vi "Test DI and DO.vi"() -> ()   [LabVIEW 2013]
uses:
  SLL DAQ Engine/Software/Source Code/Sub VIs/DAQ Engine/Controls/SLL DE List of Digital Inputs.ctl
  SLL DAQ Engine/Software/Source Code/Sub VIs/DAQ Engine/Controls/SLL DE List of Digital Outputs.ctl
  SLL DAQ Engine/Software/Source Code/Sub VIs/DAQ Engine/Controls/SLL DE DI Global Options.ctl
  SLL DAQ Engine/Software/Source Code/Sub VIs/DAQ Engine/Controls/SLL DE DO Global Options.ctl
panel:
  out "DO Channel Name":T1
  out "String":string
  in  "PC_ACK_Read_Tags":dbl
  in  "Invalid_SNo":dbl
  in  "Station_No_Start_Stop_Test":dbl
  in  "Start_Test":dbl
  in  "Rerun":dbl
  in  "Station_Number":dbl
  in  "Test_Result":dbl
  in  "Serial_Flange_Size":string
  in  "Serial_Displacement_Size":dbl
  in  "Serial_Adapter_Size":dbl
  in  "New_Serial":dbl
  in  "Scan_Trigger":dbl
  in  "Stop_Test":dbl
  in  "Task_Available_for_Robot":dbl
  in  "Robot_Available":dbl
  in  "DI Array":bool[](array[boolean])=[FALSE, FALSE, FALSE, FALSE, FALSE, FALSE, FALSE, FALSE, FALSE, FALSE, FALSE, FALSE, FALSE, FALSE, FALSE, FALSE, FALSE, FALSE, FALSE, FALSE, FALSE, FALSE, FALSE, FALSE, FALSE, FALSE, FALSE, FALSE]
  in  "DI Channel Name Array":T2[](array[typedef])=[enum."STATION1_START", enum."STATION1_STOP", enum."STATION1_CLAMPED", enum."STATION1_TC_PASS", enum."STATION1_TC_FAIL", enum."STATION1_TTA", enum."STATION1_TTB", enum."STATION2_START", enum."STATION2_STOP", enum."STATION2_CLAMPED", enum."STATION2_TC_PASS", enum."STATION2_TC_FAIL", enum."STATION2_TTA", enum."STATION2_TTB", enum."STATION3_START", enum."STATION3_STOP", enum."STATION3_CLAMPED", enum."STATION3_TC_PASS", enum."STATION3_TC_FAIL", enum."STATION3_TTA", enum."STATION3_TTB", enum."STATION4_START", enum."STATION4_STOP", enum."STATION4_CLAMPED", enum."STATION4_TC_PASS", enum."STATION4_TC_FAIL", enum."STATION4_TTA", enum."STATION4_TTB"]
  out "DO Channel Name Array":T1[](array[typedef])=[enum."STATION1_START TEST", enum."STATION1_STOP TEST", enum."STATION1_LIGHT1", enum."STATION1_LIGHT2", enum."STATION1_LIGHT3", enum."STATION1_SELECT_TEST", enum."STATION2_START TEST", enum."STATION2_STOP TEST", enum."STATION2_LIGHT1", enum."STATION2_LIGHT2", enum."STATION2_LIGHT3", enum."STATION2_SELECT_TEST", enum."STATION3_START TEST", enum."STATION3_STOP TEST", enum."STATION3_LIGHT1", enum."STATION3_LIGHT2", enum."STATION3_LIGHT3", enum."STATION3_SELECT_TEST", enum."STATION4_START TEST", enum."STATION4_STOP TEST", enum."STATION4_LIGHT1", enum."STATION4_LIGHT2", enum."STATION4_LIGHT3", enum."STATION4_SELECT_TEST"]
  out "DO Status":bool[](array[boolean])
  out "error out":errorcluster
  in  "error in":errorcluster
  in  "DI Channel Name":T2
  in  "stop":bool
  # "Simulation VI to send DI Status and reads the DO output"
  # "Write Tags\nPC Writes to PLC\nPLC can only read these tags"
  # "Read Tags\nPC Reads from PLC"
  # "Test Type1: TTA:1, TTB: 0;\nTest Type2: TTA:0, TTB: 1;\nTest Type3: TTA:1, TTB: 1;\nTest Type4: TTA:0, TTB: 0;"
  # "IDLE : \t\t100\nTest Running:\t 010\nPass\t\t110\nFail\t\t101"
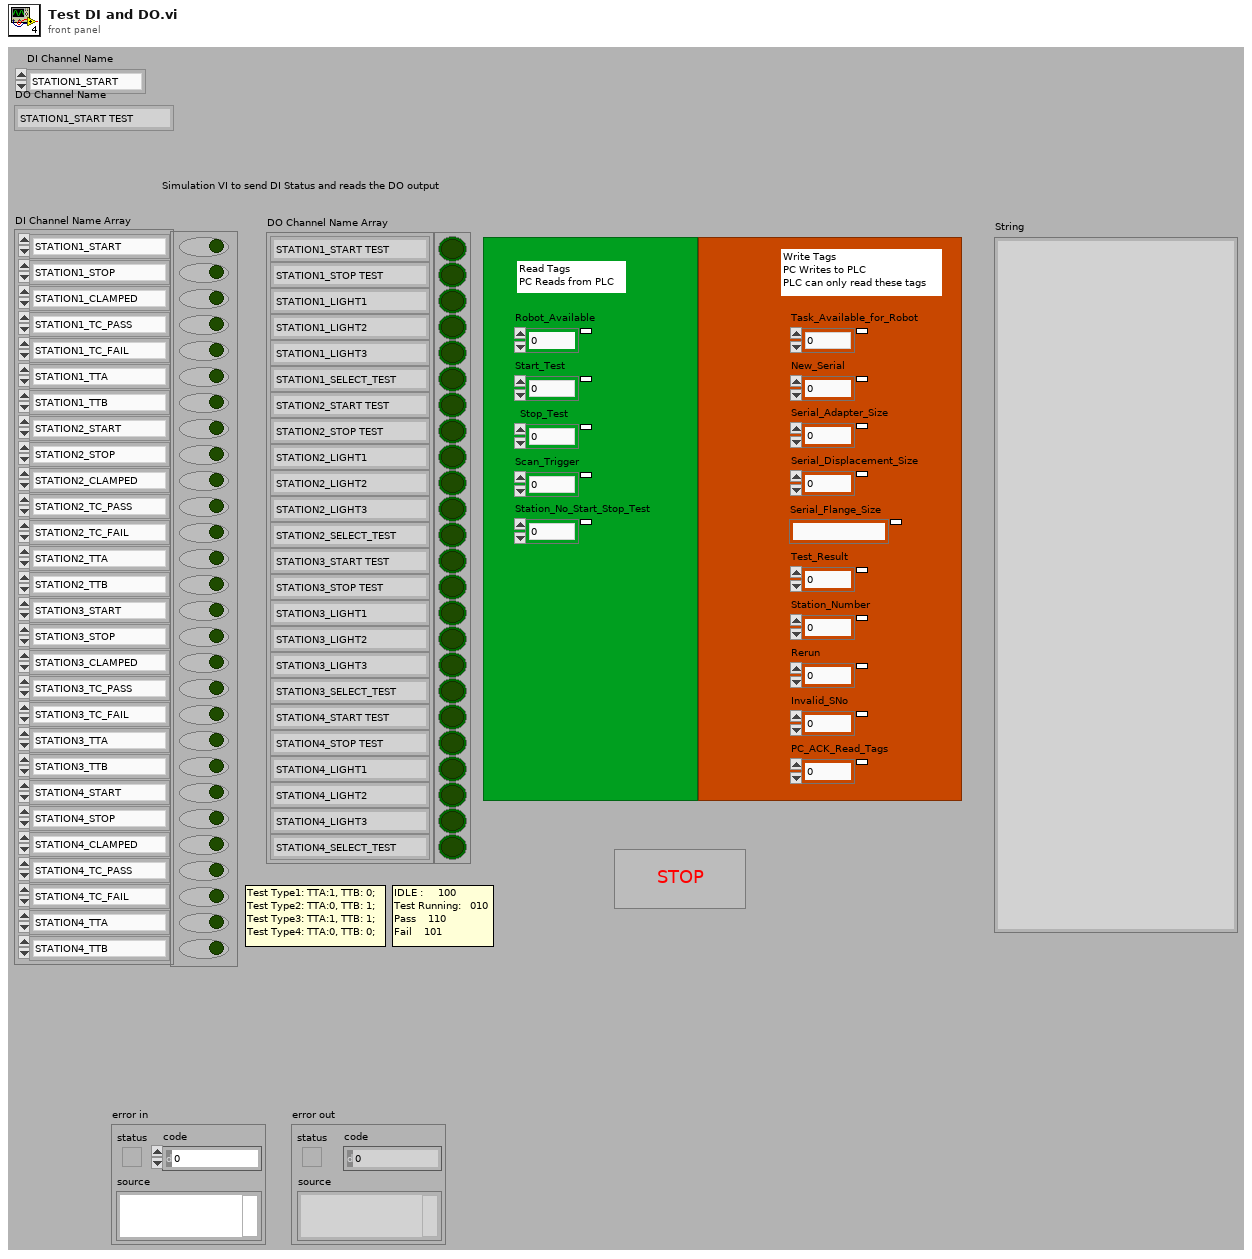
[diagram p1: front panel]
types:
  T1 = typedef "SLL DE List of Digital Outputs.ctl" = enum16{"STATION1_START TEST", "STATION1_STOP TEST", "STATION1_LIGHT1", "STATION1_LIGHT2", "STATION1_LIGHT3", "STATION1_SELECT_TEST", "STATION2_START TEST", "STATION2_STOP TEST", "STATION2_LIGHT1", "STATION2_LIGHT2", "STATION2_LIGHT3", "STATION2_SELECT_TEST", "STATION3_START TEST", "STATION3_STOP TEST", "STATION3_LIGHT1", "STATION3_LIGHT2", "STATION3_LIGHT3", "STATION3_SELECT_TEST", "STATION4_START TEST", "STATION4_STOP TEST", "STATION4_LIGHT1", "STATION4_LIGHT2", "STATION4_LIGHT3", "STATION4_SELECT_TEST"}
  T2 = typedef "SLL DE List of Digital Inputs.ctl" = enum16{"STATION1_START", "STATION1_STOP", "STATION1_CLAMPED", "STATION1_TC_PASS", "STATION1_TC_FAIL", "STATION1_TTA", "STATION1_TTB", "STATION2_START", "STATION2_STOP", "STATION2_CLAMPED", "STATION2_TC_PASS", "STATION2_TC_FAIL", "STATION2_TTA", "STATION2_TTB", "STATION3_START", "STATION3_STOP", "STATION3_CLAMPED", "STATION3_TC_PASS", "STATION3_TC_FAIL", "STATION3_TTA", "STATION3_TTB", "STATION4_START", "STATION4_STOP", "STATION4_CLAMPED", "STATION4_TC_PASS", "STATION4_TC_FAIL", "STATION4_TTA", "STATION4_TTB"}
  T3 = enum32{"No PSP", "Read", "Write", "Write & Read"}
  T4 = typedef "SLL DE DO Global Options.ctl" = enum16{"Init", "Write Line", "Write Array", "Write Full Status", "Read Line", "Read Array", "Read Full Status", "Restart DO", "Send to Safe Mode", "Stop DO"}
  T5 = typedef "SLL DE DI Global Options.ctl" = enum16{"Init", "Write Line", "Write Array", "Read Line", "Read Array", "Read Full Status", "Write Full Status"}
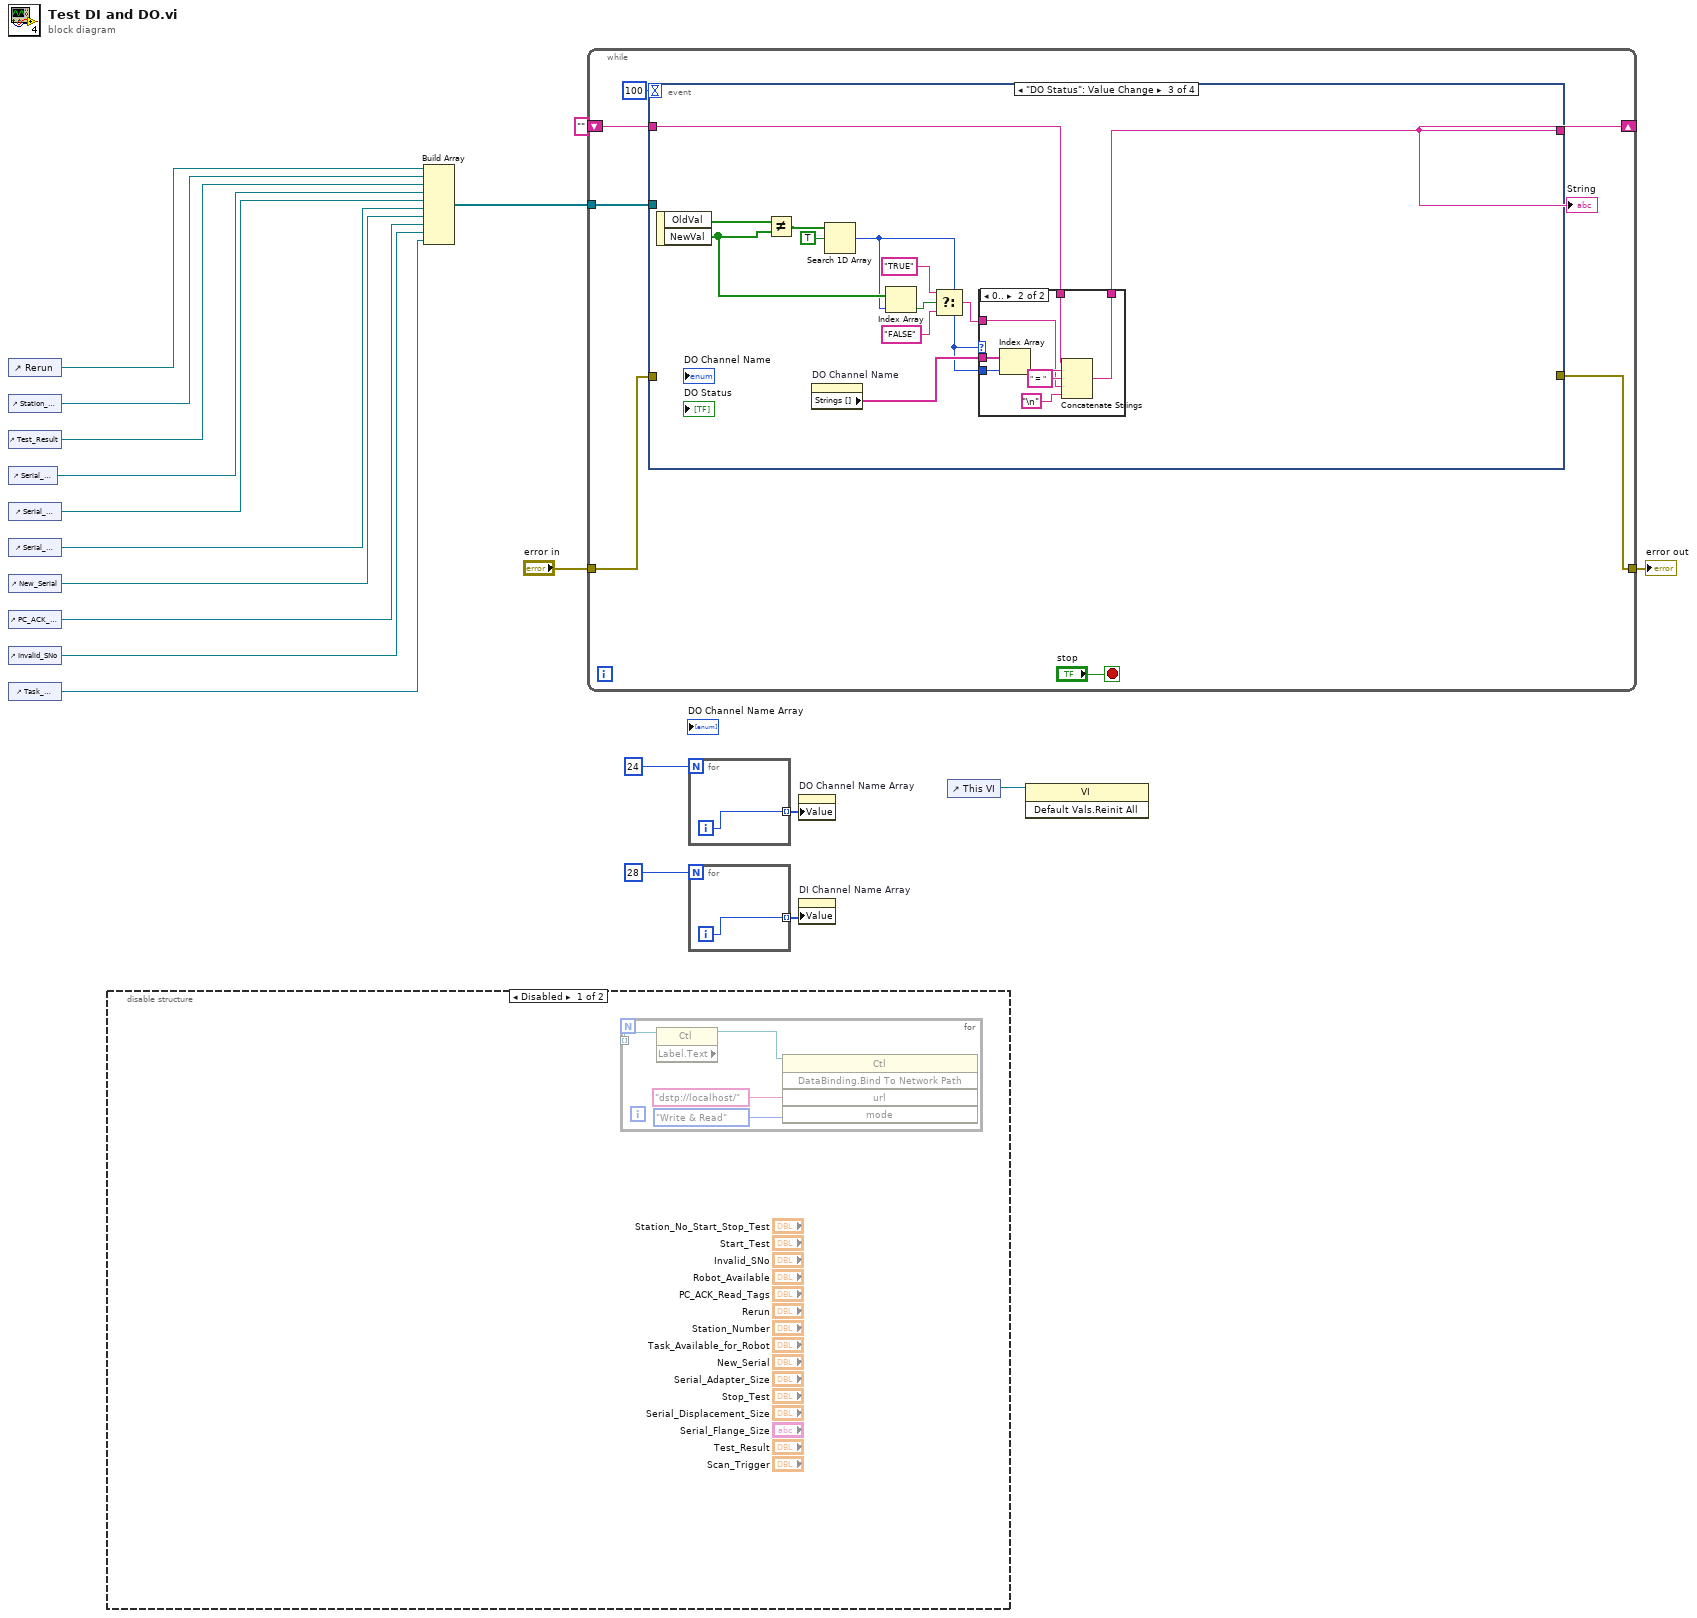
[diagram p0: block diagram]
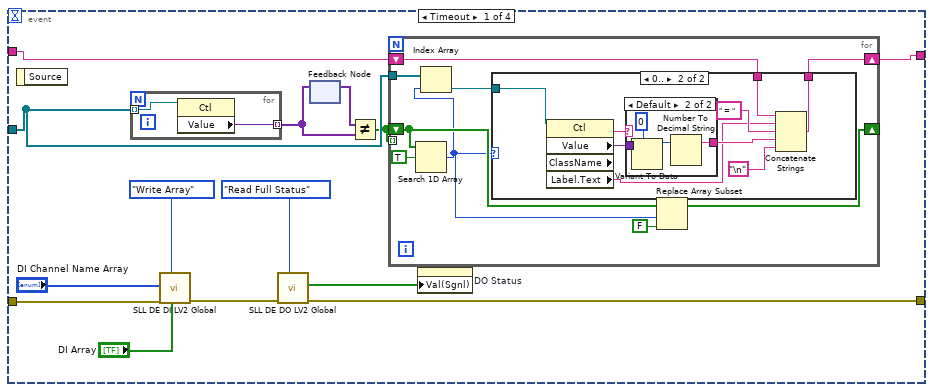
[diagram p3: hidden frame]
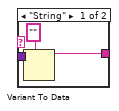
[diagram p5: hidden frame]
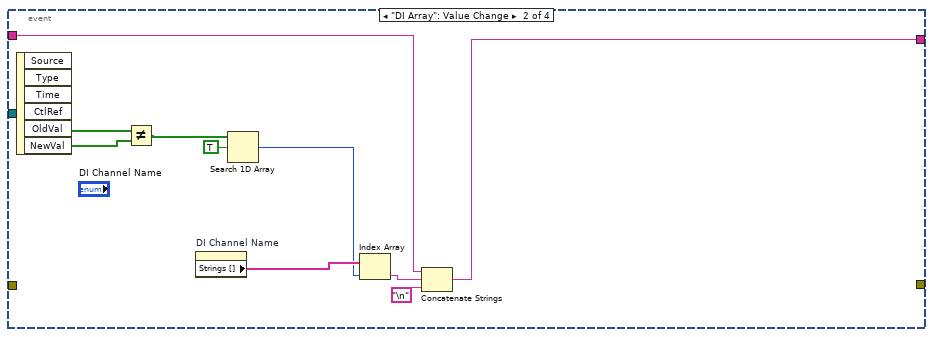
[diagram p6: hidden frame]
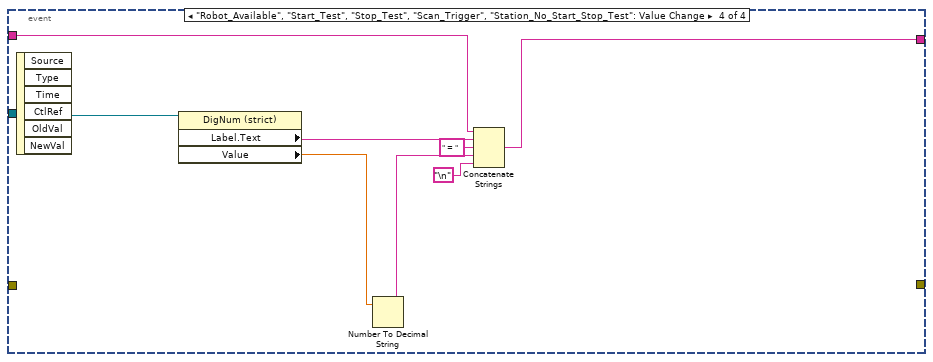
[diagram p8: hidden frame]
diagram:
  n1 = control-ref of="Rerun"() -> (w2:refnum<vi>)
  n2 = control-ref of="Station_Number"() -> (w3:refnum<vi>)
  n3 = control-ref of="Test_Result"() -> (w4:refnum<vi>)
  n4 = control-ref of="Serial_Flange_Size"() -> (w5:refnum<vi>)
  n5 = control-ref of="Serial_Displacement_Size"() -> (w6:refnum<vi>)
  n6 = control-ref of="Serial_Adapter_Size"() -> (w7:refnum<vi>)
  n7 = control-ref of="New_Serial"() -> (w8:refnum<vi>)
  n8 = control-ref of="PC_ACK_Read_Tags"() -> (w9:refnum<vi>)
  n9 = control-ref of="Invalid_SNo"() -> (w10:refnum<vi>)
  n10 = control-ref of="Task_Available_for_Robot"() -> (w11:refnum<vi>)
  n11 = disable-structure shown="Disabled" {
    frame Disabled {
      n12 = for {
        tunnel: [w24] -> w20 mode=indexing
        n13 = property class="Ctl" props=["Label", "Text"](reference=w24) -> (reference out=w21:refnum<vi>)  [unwired: 1 in, 2 out]
        n14 = invoke on="Invoke Node" class="Ctl" method="DataBinding.Bind To Network Path"(reference=w21, "url"="dstp://localhost/" ("URL"), "mode"=T3."Write & Read" ("Mode")) -> ()  [unwired: 2 in, 5 out]
      }
    }
    frame Enabled {
    }
  }
  n15 = Build Array(w2, w3, w4, w5, w6, w7, w8, w9, w10, w11) -> (w1:refnum<vi>[])
  n16 = while {
    tunnel: "error in" -> [w27]
    tunnel: [w26] -> w19
    shift-right: [w30] -> _
    shift-left: "" -> [w28]
    tunnel: w1 -> [w25]
    stop <- "stop" stop-if-true
    n17 = event shown="[2] \"DO Status\": Value Change" {
      selector: _ -> [_ _ _ _]
      dyn-events: _ -> [_ _ _ _]
      timeout: 100 -> [_ _ _ _]
      tunnel: [w33 w75 w92 w110] -> w30
      tunnel: w28 -> [w34 w74 w91 w111]
      tunnel: w27 -> [w39 _ _ _]
      tunnel: [w38 _ _ _] -> w26
      tunnel: w25 -> [w35 _ _ _]
      event Timeout {
        n18 = event-data() -> ()  [unwired: 1 in, 1 out]
        n19 = for {
          tunnel: w35 -> [w73] mode=indexing
          tunnel: [w72] -> w36 mode=indexing
          n20 = property class="Ctl"(reference=w73) -> ("Value"=w72:variant)  [unwired: 1 in, 2 out]
        }
        n21 = call "SLL DE DI LV2 Global.vi"("DI State Array"="DI Array", "Option"=SLL_DE_DI_Global_Options."Write Array", "error in (no error)"=w39, "DI Channel Name Array"="DI Channel Name Array") -> ("error out"=w44:errorcluster)  [unwired: 4 in, 3 out]
        n22 = call "SLL DE DO LV2 Global.vi"("DO Option"=SLL_DE_DO_Global_Options."Read Full Status", "Error In"=w44) -> ("error out"=w38:errorcluster, "Digital Array Status"=w45:bool[])  [unwired: 6 in, 2 out]
        n23 = feedback-in #1(w36) -> ()
        n24 = feedback #1() -> (w37:variant[])  [unwired: 1 in]
        n25 = Not Equal?(x=w37, y=w36) -> (x != y?=w32:bool[])
        n26 = for {
          tunnel: w35 -> [w53]
          shift-right: [w48] -> _
          shift-left: w32 -> [w49]
          tunnel: w32 -> [_] mode=indexing
          shift-right: [w51] -> w33
          shift-left: w34 -> [w52]
          n27 = Search 1D Array(1D array=w49, element=TRUE) -> (index of element=w47:i32)  [unwired: 1 in]
          n28 = Index Array(array=w53, index=w47) -> (element=w50:refnum<vi>)
          n29 = case shown="0.." w47 {
            tunnel: [w55 w63] -> w51
            tunnel: w52 -> [w55 w62]
            tunnel: w50 -> [_ w59]
            frame -1, Default {
            }
            frame 0.. {
              n30 = property class="Ctl"(reference=w59) -> ("Value"=w61:variant, "ClassName"=w58:string, "Label.Text"=w56:string)  [unwired: 1 in, 2 out]
              n31 = case shown="Default" w58 {
                tunnel: w61 -> [w66 w70]
                tunnel: [w65 w68] -> w60
                frame "String" {
                  n32 = Variant To Data(type="" ("concatenated string"), Variant=w66) -> (data=w65:string)  [unwired: 1 in, 1 out]
                }
                frame Default {
                  n33 = Variant To Data(type=0 ("concatenated string"), Variant=w70) -> (data=w69:i32)  [unwired: 1 in, 1 out]
                  n34 = Number To Decimal String(number=w69) -> (decimal integer string=w68:string)  [unwired: 1 in]
                }
              }
              n35 = Concatenate Strings(w62, w56, " = " ("string"), w60, "\n") -> (w63:string)
            }
          }
          n36 = Replace Array Subset(array=w49, new element=FALSE ("new element/subarray"), index=w47) -> (w48:bool[])
        }
        n37 = property on="DO Status" class="Arr (strict)"("Val(Sgnl)"=w45) -> ()  [unwired: 2 in, 2 out]
      }
      event "DI Array": Value Change {
        n38 = event-data() -> ("OldVal"=w83:bool[], "NewVal"=w82:bool[])  [unwired: 1 in, 4 out]
        n39 = Not Equal?(x=w83, y=w82) -> (x != y?=w81:bool[])
        n40 = property on="DI Channel Name" class="Enum (strict)"() -> ("Strings []"=w79:string[])  [unwired: 2 in, 2 out]
        n41 = Search 1D Array(1D array=w81, element=TRUE) -> (index of element=w78:i32)  [unwired: 1 in]
        n42 = Index Array(array=w79, index=w78) -> (element=w76:string)
        n43 = Concatenate Strings(w74, w76, "\n") -> (w75:string)
      }
      event "DO Status": Value Change {
        n44 = event-data() -> ("OldVal"=w95:bool[], "NewVal"=w89:bool[])  [unwired: 1 in]
        n45 = Not Equal?(x=w95, y=w89) -> (x != y?=w94:bool[])
        n46 = property on="DO Channel Name" class="Enum (strict)"() -> ("Strings []"=w90:string[])  [unwired: 2 in, 2 out]
        n47 = Search 1D Array(1D array=w94, element=TRUE) -> (index of element=w88:i32)  [unwired: 1 in]
        n48 = Index Array(array=w89, index=w88) -> (element=w87:bool)
        n49 = Select(t="TRUE", s=w87, f="FALSE") -> (s? t:f=w84:string)
        n50 = case shown="0.." w88 {
          tunnel: w88 -> [_ w104]
          tunnel: [w96 w101] -> w92
          tunnel: w90 -> [_ w100]
          tunnel: w91 -> [w96 w99]
          tunnel: w84 -> [_ w97]
          frame -1, Default {
          }
          frame 0.. {
            n51 = Index Array(array=w100, index=w104) -> (element=w102:string)
            n52 = Concatenate Strings(w99, w102, " = " ("string"), w97, "\n") -> (w101:string)
          }
        }
      }
      event "Robot_Available", "Start_Test", "Stop_Test", "Scan_Trigger", "Station_No_Start_Stop_Test": Value Change {
        n53 = event-data() -> ("CtlRef"=w112:refnum<vi>)  [unwired: 1 in, 5 out]
        n54 = property class="DigNum (strict)"(reference=w112) -> ("Label.Text"=w109:string, "Value"=w108:dbl)  [unwired: 1 in, 2 out]
        n55 = Number To Decimal String(number=w108) -> (decimal integer string=w107:string)  [unwired: 1 in]
        n56 = Concatenate Strings(w111, w109, " = " ("string"), w107, "\n") -> (w110:string)
      }
    }
    "String" <- w30
  }
  "error out" <- w19
  n57 = for {
    N: 24 -> [_]
    tunnel: [w113] -> w17 mode=indexing
    i -> [w113]
  }
  n58 = for {
    N: 28 -> [_]
    tunnel: [w114] -> w14 mode=indexing
    i -> [w114]
  }
  n59 = property on="DO Channel Name Array" class="Arr (strict)"("Value"=w17) -> ()  [unwired: 2 in, 2 out]
  n60 = property on="DI Channel Name Array" class="Arr (strict)"("Value"=w14) -> ()  [unwired: 2 in, 2 out]
  n61 = control-ref of="This VI"() -> (w13:refnum<vi>)
  n62 = invoke class="VI" method="Default Vals.Reinit All"(reference=w13) -> ()  [unwired: 2 in, 3 out]
